vi "Avg_Example_IMAQ.vi"() -> ()   [LabVIEW 2019]
doc: "This example shows how to continously compute and show an averaged image.\nHere the camera class is operated in sequence mode and the required number of images also defines the number of images that will be averaged\nIt is a good starting point for writing own applications.\nBut it will not be fail save, i.e. doesnt react on errors, just handles them forward to the end\n\nUsage:\nSelect your required image count you want to average over before you start the program.\nOnce started, the camera class will be initialized and image record will start automatically.\nInside the acquisition loop the program will record the image sequence.\nThen it calculates the average image and shows it.\nBy using the ROI parameters you can crop the image to select certain regions\n\nBy clicking Quit Application the record will stop and will force an exit of the camera class"
uses:
  camera/Camera.lvclass
panel:
  out "rawImage":u16[][](array[numeric])
  out "Image":T1(plugin-control)
  in  "data_format":T2(ring)=enum."Mono16"
  out "Recorded Images":u32
  in  "Quit":bool
  in  "cropY1":u64=2 min=2 max=1040 step=1
  in  "cropX1":u64=2 min=2 max=1392 step=1
  in  "cropY0":u64=1 min=1 max=1039 step=1
  in  "cropX0":u64=1 min=1 max=1391 step=1
  out "Image Height":u64
  out "Image Width":u64
  in  "dwImgCount":u32=10 caption="Required Number of Images" max=4023
  out "Error":errorcluster {"code" format="%x"}
  # "This example shows how to continously compute and show an averaged image.\nHere the camera class is operated in sequence mode and the required number of images also defines the number of images that will be averaged\nIt is a good starting point for writing own applications.\nBut it will not be fail save, i.e. doesnt react on errors, just handles them forward to the end\n\nUsage:\nSelect your required image count you want to average over before you start the program.\nOnce started, the camera class will be initialized and image record will start automatically.\nInside the acquisition loop the program will record the image sequence.\nThen it calculates the average image and shows it.\nBy using the crop parameters you can crop the image to select certain regions\n\nBy clicking Quit Application the record will stop and will force an exit of the camera class"
  # "pco.labview"
  # "Camera Setup"
  # "Recording Control"
  # "Parameters for image readout"
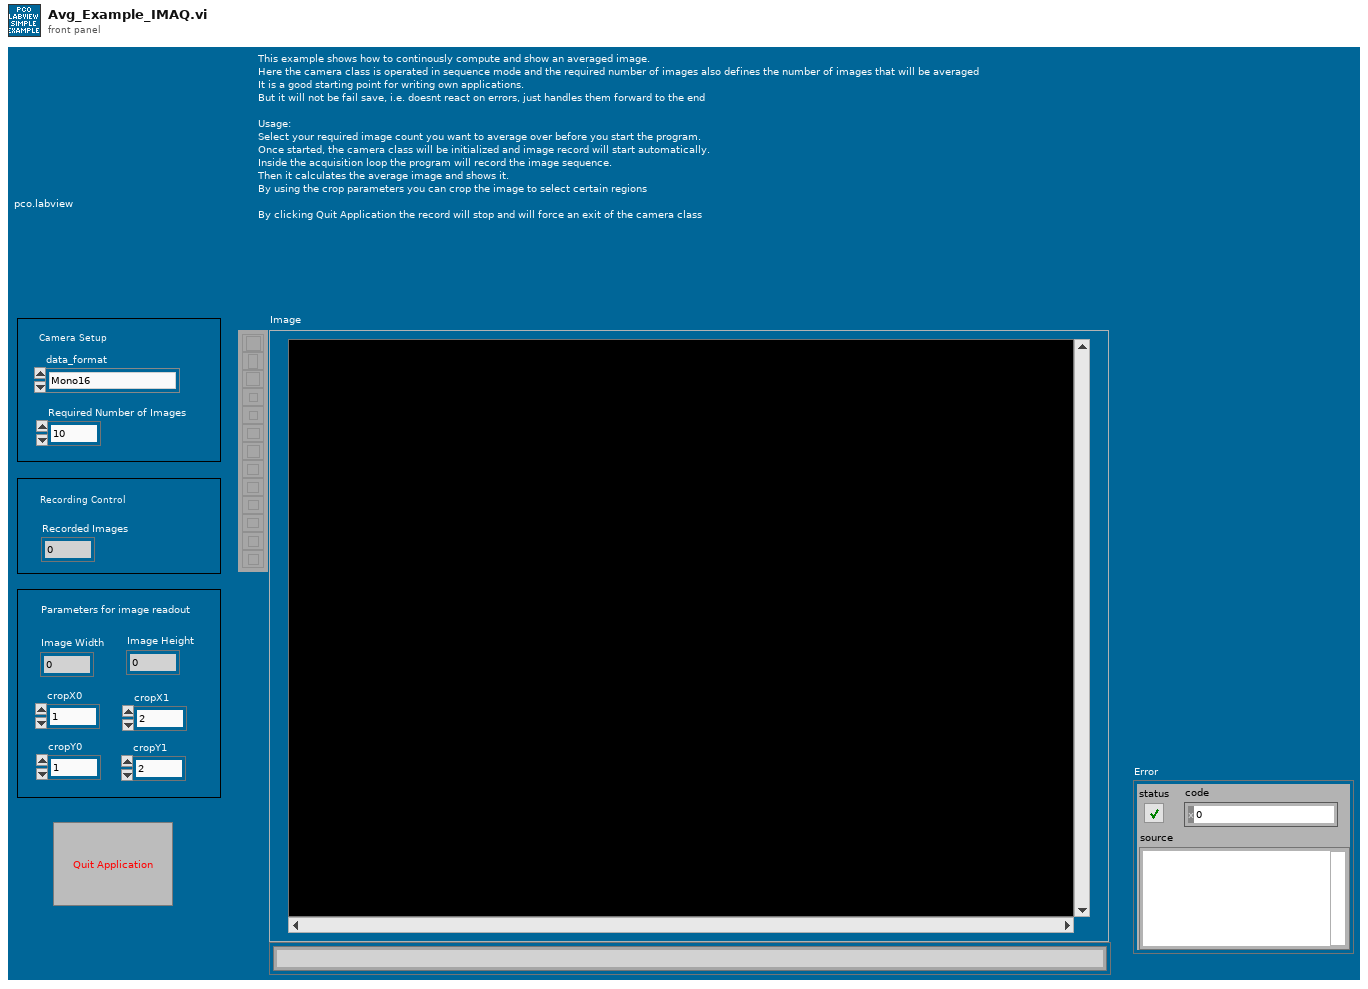
[diagram p1: front panel]
types:
  T1 = typedef "IMAQ Image.ctl" = refnum<image>
  T2 = enum16{"Undefined", "Mono8", "Mono16", "BGRA8", "RGBA8", "BGRA16", "RGBA16", "CompressedMono8"}
  T3 = enum8{"Enabled", "Disabled", "Disabled and Grayed Out"}
  T4 = enum16{"sequence", "sequence non blocking", "ring buffer", "fifo", "tif", "multitif", "pcoraw", "b16", "dicom", "multidicom", "camram_ring", "camram_segment"}
  T5 = cluster{"serial":u32, "type":u16, "sub_type":u16, "interface_type":u16, "bit_resolution":u16, "min_exposure_time_s":dbl, "max_exposure_time_s":dbl, "min_exposure_step_s":dbl, "min_delay_time_s":dbl, "max_delay_time_s":dbl, "min_delay_step_s":dbl, "min_width":u64, "min_height":u64, "max_width":u64, "max_height":u64, "roi_step_horz":u64, "roi_step_vert":u64, "roi_symmetric_horz":bool, "roi_symmetric_vert":bool, "has_timestamp_mode":bool, "has_timestamp_mode_ascii_only":bool, "pixelrate_vec":u32[], "conversion_factor_vec":sgl[], "has_trigger_mode_extexpctrl":bool, "has_acquire_mode":bool, "has_ext_acquire_mode":bool, "has_metadata_mode":bool, "has_ram":bool, "binning_horz_vec":u16[], "binning_vert_vec":u16[], "has_average_binning":bool, "pixel_format_vec":u32[]}
  T6 = typedef "Image Type" = u32
  T7 = typedef "Camera.lvclass/binning.ctl" = cluster{"vert":u16, "horz":u16, "mode":u16}
  T8 = cluster{"exposure_time_s":dbl, "delay_time_s":dbl, "roi":cluster{"x0":u64, "y0":u64, "x1":u64, "y1":u64}, "timestamp_mode":u16, "pixelrate":u32, "conversion_factor":sgl, "trigger_mode":u16, "acquire_mode":u16, "acquire_sequence_number":u32, "metadata_mode":u16, "noisefilter_mode":u16, "pixel_format":u32, "binning":T7, "auto_exposure":cluster{"region":u16, "min_exposure_s":dbl, "max_exposure_s":dbl}}
  T9 = cluster{"Plane 4 (alpha)":u16, "Plane 1 (Red)":u16, "Plane 2 (Green)":u16, "Plane 3 (Blue)":u16}[][]
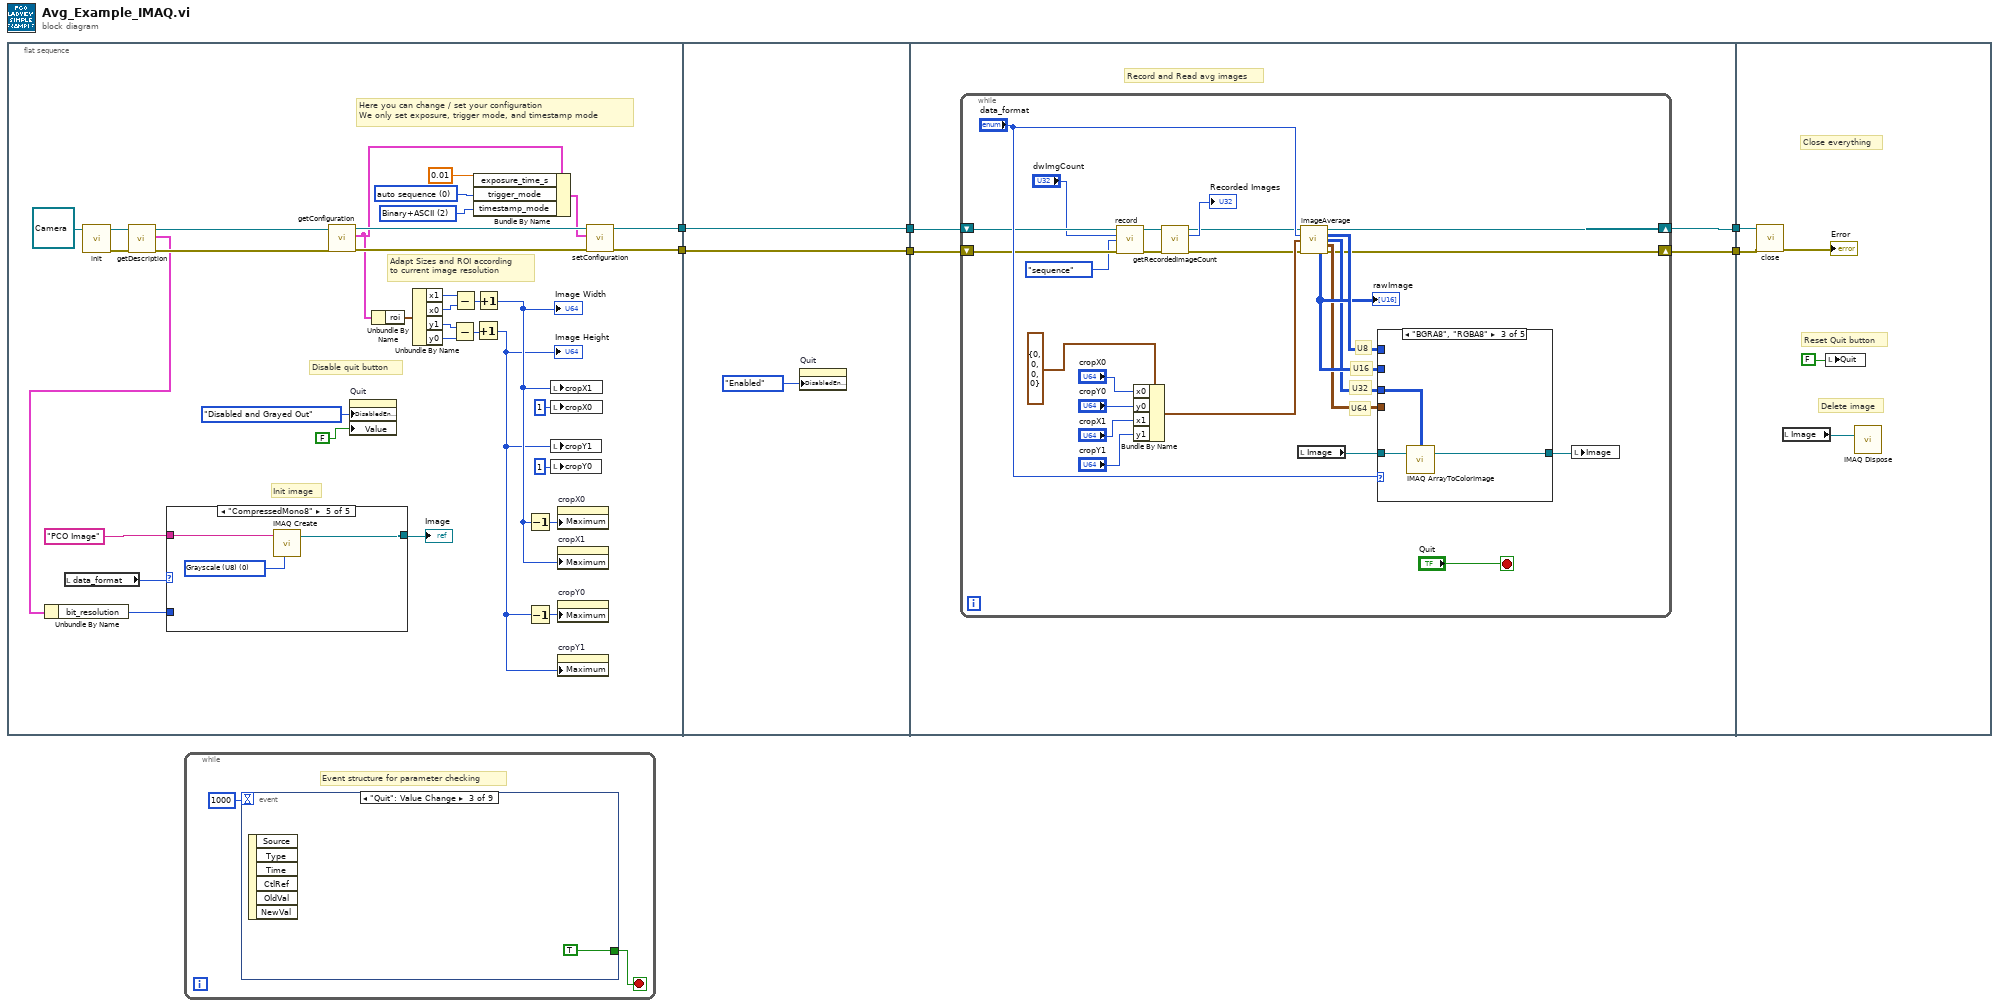
[diagram p0: block diagram]
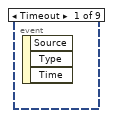
[diagram p2: hidden frame]
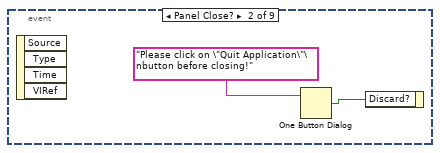
[diagram p3: hidden frame]
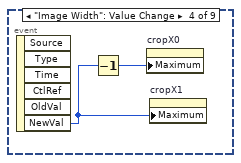
[diagram p4: hidden frame]
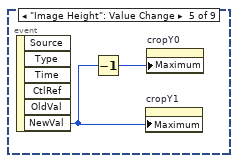
[diagram p5: hidden frame]
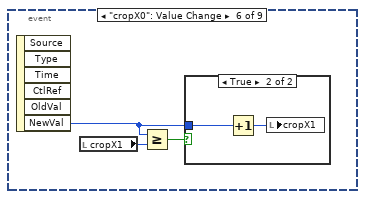
[diagram p6: hidden frame]
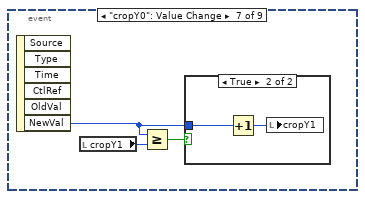
[diagram p8: hidden frame]
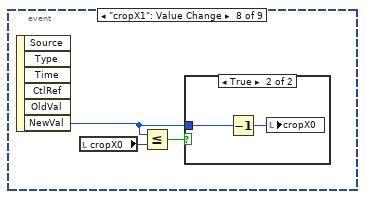
[diagram p10: hidden frame]
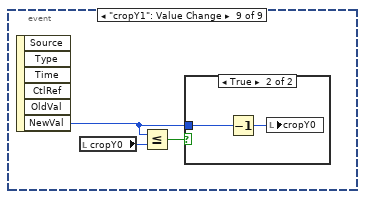
[diagram p12: hidden frame]
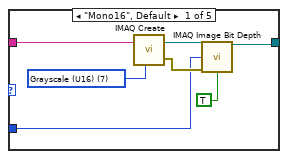
[diagram p14: hidden frame]
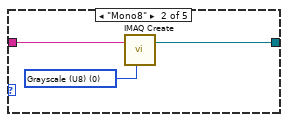
[diagram p15: hidden frame]
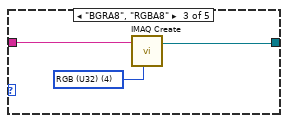
[diagram p16: hidden frame]
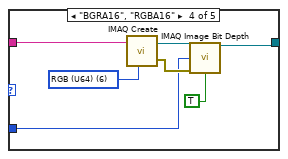
[diagram p17: hidden frame]
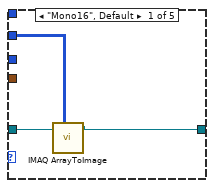
[diagram p18: hidden frame]
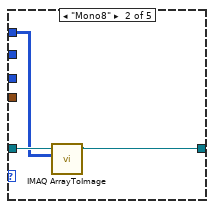
[diagram p19: hidden frame]
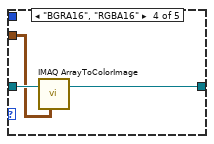
[diagram p20: hidden frame]
diagram:
  n1 = flat-sequence {
    tunnel: [w15] -> w6
    tunnel: [w14] -> w5
    tunnel: w6 -> [w65]
    tunnel: w5 -> [w64]
    tunnel: [w65] -> w4
    tunnel: [w64] -> w3
    tunnel: [w70] -> w2
    tunnel: [w69] -> w1
    tunnel: w3 -> [w68]
    tunnel: w4 -> [w67]
    tunnel: w2 -> [w113]
    tunnel: w1 -> [w112]
    frame #0 {
      w21 = u16 2 items=["OFF", "Binary", "Binary+ASCII", "ASCII"] ("TimestampMode")
      w39 = u16 0 items=["auto sequence"=0, "software trigger"=1, "external exposure start & software trigger"=2, "external exposure control"=3, "external synchronized"=4, "fast external exposure control"=5, "external CDS control"=6, "slow external exposure control"=7, "external synchronized HDSDI"=258] ("TriggerMode")
      # "Here you can change / set your configuration\nWe only set exposure, trigger mode, and timestamp mode"
      # "Init image"
      # "Adapt Sizes and ROI according\nto current image resolution"
      # "Disable quit button"
      n2 = local read "data_format"() -> (w18:T2)
      n3 = call-dynamic "init.vi"("Camera in"=refnum<class "Camera.lvclass"> refnum ("PCOCamera in")) -> ("Camera out"=w12:refnum<class "Camera.lvclass">, "error out"=w13:errorcluster)  [unwired: 8 in]
      n4 = call-dynamic "getDescription.vi"("error in (no error)"=w13, "Camera in"=w12) -> ("error out"=w10:errorcluster, "description"=w9:T5, "Camera out"=w11:refnum<class "Camera.lvclass">)  [unwired: 7 in]
      n5 = Unbundle By Name(w9) -> ("bit_resolution"=w8:u16)
      n6 = case shown="\"CompressedMono8\"" w18 {
        tunnel: "PCO Image" ("Image Name") -> [w46 w50 w52 w59 w62]
        tunnel: [w42 w48 w51 w55 w61] -> w17
        tunnel: w8 -> [w41 _ _ w54 _]
        frame "Mono16", Default {
          w47 = T6 7 items=["Grayscale (U8)", "Grayscale (I16)", "Grayscale (SGL)", "Complex (CSG)", "RGB (U32)", "HSL (U32)", "RGB (U64)", "Grayscale (U16)"] ("Image Type")
          n7 = call "IMAQ Create"("Image Name"=w46, "Image Type"=w47) -> ("New Image"=w44:T1, "error out"=w43:errorcluster)  [unwired: 3 in]
          n8 = call "IMAQ Image Bit Depth"("Image"=w44, "Bit Depth (0)"=w41, "error in (no error)"=w43, "Get/Set Bit Depth? (Set)"=TRUE) -> ("Image Out"=w42:T1)  [unwired: 9 in, 2 out]
        }
        frame "Mono8" {
          w49 = T6 0 items=["Grayscale (U8)", "Grayscale (I16)", "Grayscale (SGL)", "Complex (CSG)", "RGB (U32)", "HSL (U32)", "RGB (U64)", "Grayscale (U16)"] ("Image Type")
          n9 = call "IMAQ Create"("Image Name"=w50, "Image Type"=w49) -> ("New Image"=w48:T1)  [unwired: 3 in, 1 out]
        }
        frame "BGRA8", "RGBA8" {
          w53 = T6 4 items=["Grayscale (U8)", "Grayscale (I16)", "Grayscale (SGL)", "Complex (CSG)", "RGB (U32)", "HSL (U32)", "RGB (U64)", "Grayscale (U16)"] ("Image Type")
          n10 = call "IMAQ Create"("Image Name"=w52, "Image Type"=w53) -> ("New Image"=w51:T1)  [unwired: 3 in, 1 out]
        }
        frame "BGRA16", "RGBA16" {
          w60 = T6 6 items=["Grayscale (U8)", "Grayscale (I16)", "Grayscale (SGL)", "Complex (CSG)", "RGB (U32)", "HSL (U32)", "RGB (U64)", "Grayscale (U16)"] ("Image Type")
          n11 = call "IMAQ Create"("Image Name"=w59, "Image Type"=w60) -> ("New Image"=w57:T1, "error out"=w56:errorcluster)  [unwired: 3 in]
          n12 = call "IMAQ Image Bit Depth"("Image"=w57, "Bit Depth (0)"=w54, "error in (no error)"=w56, "Get/Set Bit Depth? (Set)"=TRUE) -> ("Image Out"=w55:T1)  [unwired: 9 in, 2 out]
        }
        frame "CompressedMono8" {
          w63 = T6 0 items=["Grayscale (U8)", "Grayscale (I16)", "Grayscale (SGL)", "Complex (CSG)", "RGB (U32)", "HSL (U32)", "RGB (U64)", "Grayscale (U16)"] ("Image Type")
          n13 = call "IMAQ Create"("Image Name"=w62, "Image Type"=w63) -> ("New Image"=w61:T1)  [unwired: 3 in, 1 out]
        }
      }
      "Image" <- w17
      n14 = call-dynamic "getConfiguration.vi"("error in (no error)"=w10, "Camera in"=w11) -> ("error out"=w37:errorcluster, "configuration"=w31:T8, "Camera out"=w38:refnum<class "Camera.lvclass">)  [unwired: 7 in]
      n15 = property on="Quit" class="Bool (strict)"("DisabledEnum"=T3."Disabled and Grayed Out" ("Disabled"), "Value"=FALSE ("Stop")) -> ()  [unwired: 2 in, 2 out]
      n16 = Unbundle By Name(w31) -> ("roi"=w30:cluster{"x0":u64, "y0":u64, "x1":u64, "y1":u64})
      n17 = Unbundle By Name(w30) -> ("x1"=w28:u64, "x0"=w29:u64, "y1"=w26:u64, "y0"=w27:u64)
      n18 = Subtract(x=w26, y=w27) -> (x-y=w24:u64)
      n19 = Subtract(x=w28, y=w29) -> (x-y=w25:u64)
      n20 = Bundle By Name(cluster=w31, "exposure_time_s"=0.01, "trigger_mode"=w39, "timestamp_mode"=w21) -> (w36:T8)
      n21 = Increment(x=w24) -> (x+1=w22:u64)
      "Image Height" <- w22
      n22 = Increment(x=w25) -> (x+1=w23:u64)
      "Image Width" <- w23
      n23 = Decrement(x=w23) -> (x-1=w33:u64)
      n24 = Decrement(x=w22) -> (x-1=w32:u64)
      n25 = local write "cropX1"(w23) -> ()
      n26 = local write "cropX0"(u64 1 ("roiY0")) -> ()
      n27 = local write "cropY1"(w22) -> ()
      n28 = local write "cropY0"(u64 1 ("roiY0")) -> ()
      n29 = property on="cropX0" class="DigNum (strict)"("Maximum"=w33) -> ()  [unwired: 2 in, 2 out]
      n30 = property on="cropX1" class="DigNum (strict)"("Maximum"=w23) -> ()  [unwired: 2 in, 2 out]
      n31 = property on="cropY0" class="DigNum (strict)"("Maximum"=w32) -> ()  [unwired: 2 in, 2 out]
      n32 = property on="cropY1" class="DigNum (strict)"("Maximum"=w22) -> ()  [unwired: 2 in, 2 out]
      n33 = call-dynamic "setConfiguration.vi"("error in (no error)"=w37, "configuration"=w36, "Camera in"=w38) -> ("error out"=w14:errorcluster, "Camera out"=w15:refnum<class "Camera.lvclass">)  [unwired: 7 in]
    }
    frame #1 {
      n34 = property on="Quit" class="Bool (strict)"("DisabledEnum"=T3."Enabled" ("Disabled")) -> ()  [unwired: 2 in, 2 out]
    }
    frame #2 {
      # "Record and Read avg images"
      n35 = while {
        shift-right: [w81] -> w70
        shift-left: w67 -> [w80]
        shift-right: [w72] -> w69
        shift-left: w68 -> [w79]
        stop <- "Quit" stop-if-true
        # "U64"
        # "U32"
        # "U16"
        # "U8"
        n36 = call-dynamic "record.vi"("Camera in"=w80, "num_images"="dwImgCount", "record_mode"=T4."sequence", "error in (no error)"=w79) -> ("Camera out"=w78:refnum<class "Camera.lvclass">, "error out"=w77:errorcluster)  [unwired: 10 in]
        n37 = Bundle By Name(cluster=cluster{"x0":u64, "y0":u64, "x1":u64, "y1":u64} {"x0"=0, "y0"=0, "x1"=0, "y1"=0} ("roi"), "x0"="cropX0", "y0"="cropY0", "x1"="cropX1", "y1"="cropY1") -> (w91:cluster{"x0":u64, "y0":u64, "x1":u64, "y1":u64})
        n38 = call-dynamic "getRecordedImageCount.vi"("Camera in"=w78, "error in (no error)"=w77) -> ("Camera out"=w75:refnum<class "Camera.lvclass">, "recorded_image_count"=→"Recorded Images":u32, "error out"=w74:errorcluster)  [unwired: 11 in]
        n39 = local read "Image"() -> (w85:T1)
        n40 = call-dynamic "imageAverage.vi"("Camera in"=w75, "data_format"="data_format", "crop"=w91, "error in (no error)"=w74) -> ("Camera out"=w81:refnum<class "Camera.lvclass">, "image (U8)"=w89:u8[][], "image (U32)"=w87:u32[][], "image (U64)"=w86:T9, "raw_image (U16)"=w88:u16[][], "error out"=w72:errorcluster)  [unwired: 5 in, 1 out]
        "rawImage" <- w88
        n41 = case shown="\"BGRA8\", \"RGBA8\"" "data_format" {
          tunnel: w85 -> [w98 w101 w104 w107 w110]
          tunnel: [w96 w99 w103 w105 w109] -> w84
          tunnel: w86 -> [_ _ _ w106 _]
          tunnel: w87 -> [_ _ w102 _ _]
          tunnel: w89 -> [_ w100 _ _ w108]
          tunnel: w88 -> [w97 _ _ _ _]
          frame "Mono16", Default {
            n42 = call "IMAQ ArrayToImage"("Image Pixels (U16)"=w97, "Image"=w98) -> ("Image Out"=w96:T1)  [unwired: 8 in, 1 out]
          }
          frame "Mono8" {
            n43 = call "IMAQ ArrayToImage"("Image Pixels (U8)"=w100, "Image"=w101) -> ("Image Out"=w99:T1)  [unwired: 8 in, 1 out]
          }
          frame "BGRA8", "RGBA8" {
            n44 = call "IMAQ ArrayToColorImage"("Image Pixels (U32)"=w102, "Image"=w104) -> ("Image Out"=w103:T1)  [unwired: 3 in, 1 out]
          }
          frame "BGRA16", "RGBA16" {
            n45 = call "IMAQ ArrayToColorImage"("Image"=w107, "Image Pixels (U64)"=w106) -> ("Image Out"=w105:T1)  [unwired: 3 in, 1 out]
          }
          frame "CompressedMono8" {
            n46 = call "IMAQ ArrayToImage"("Image Pixels (U8)"=w108, "Image"=w110) -> ("Image Out"=w109:T1)  [unwired: 8 in, 1 out]
          }
        }
        n47 = local write "Image"(w84) -> ()
      }
    }
    frame #3 {
      # "Delete image"
      # "Reset Quit button"
      # "Close everything"
      n48 = call-dynamic "close.vi"("error in (no error)"=w112, "Camera in"=w113) -> ("error out"=→"Error":errorcluster)  [unwired: 9 in]
      n49 = local read "Image"() -> (w111:T1)
      n50 = local write "Quit"(FALSE ("Stop")) -> ()
      n51 = call "IMAQ Dispose"("Image"=w111) -> ()  [unwired: 5 in, 1 out]
    }
  }
  n52 = while {
    stop <- w116 stop-if-true
    # "Event structure for parameter checking"
    n53 = event shown="[2] \"Quit\": Value Change" {
      selector: _ -> [_ _ _ _ _ _ _ _ _]
      dyn-events: _ -> [_ _ _ _ _ _ _ _ _]
      timeout: 1000 -> [_ _ _ _ _ _ _ _ _]
      tunnel: [_ _ TRUE _ _ _ _ _ _] -> w116
      event Timeout {
        n54 = event-data() -> ()  [unwired: 1 in, 3 out]
      }
      event Panel Close? {
        n55 = event-data() -> ()  [unwired: 1 in, 4 out]
        n56 = One Button Dialog(message="Please click on \"Quit Application\"\nbutton before closing!") -> (true=w118:bool)  [unwired: 1 in]
        n57 = event-data("Discard?"=w118) -> ()  [unwired: 1 in, 1 out]
      }
      event "Quit": Value Change {
        n58 = event-data() -> ()  [unwired: 1 in, 6 out]
      }
      event "Image Width": Value Change {
        n59 = event-data() -> ("NewVal"=w121:u64)  [unwired: 1 in, 5 out]
        n60 = Decrement(x=w121) -> (x-1=w122:u64)
        n61 = property on="cropX0" class="DigNum (strict)"("Maximum"=w122) -> ()  [unwired: 2 in, 2 out]
        n62 = property on="cropX1" class="DigNum (strict)"("Maximum"=w121) -> ()  [unwired: 2 in, 2 out]
      }
      event "Image Height": Value Change {
        n63 = event-data() -> ("NewVal"=w123:u64)  [unwired: 1 in, 5 out]
        n64 = Decrement(x=w123) -> (x-1=w124:u64)
        n65 = property on="cropY1" class="DigNum (strict)"("Maximum"=w123) -> ()  [unwired: 2 in, 2 out]
        n66 = property on="cropY0" class="DigNum (strict)"("Maximum"=w124) -> ()  [unwired: 2 in, 2 out]
      }
      event "cropX0": Value Change {
        n67 = event-data() -> ("NewVal"=w125:u64)  [unwired: 1 in, 5 out]
        n68 = local read "cropX1"() -> (w127:u64)
        n69 = Greater Or Equal?(x=w125, y=w127) -> (x >= y?=w126:bool)
        n70 = case shown="True" w126 {
          tunnel: w125 -> [_ w129]
          frame False {
          }
          frame True {
            n71 = Increment(x=w129) -> (x+1=w128:u64)
            n72 = local write "cropX1"(w128) -> ()
          }
        }
      }
      event "cropY0": Value Change {
        n73 = event-data() -> ("NewVal"=w130:u64)  [unwired: 1 in, 5 out]
        n74 = local read "cropY1"() -> (w132:u64)
        n75 = Greater Or Equal?(x=w130, y=w132) -> (x >= y?=w131:bool)
        n76 = case shown="True" w131 {
          tunnel: w130 -> [_ w134]
          frame False {
          }
          frame True {
            n77 = Increment(x=w134) -> (x+1=w133:u64)
            n78 = local write "cropY1"(w133) -> ()
          }
        }
      }
      event "cropX1": Value Change {
        n79 = event-data() -> ("NewVal"=w135:u64)  [unwired: 1 in, 5 out]
        n80 = local read "cropX0"() -> (w137:u64)
        n81 = Less Or Equal?(x=w135, y=w137) -> (x <= y?=w136:bool)
        n82 = case shown="True" w136 {
          tunnel: w135 -> [_ w139]
          frame False {
          }
          frame True {
            n83 = Decrement(x=w139) -> (x-1=w138:u64)
            n84 = local write "cropX0"(w138) -> ()
          }
        }
      }
      event "cropY1": Value Change {
        n85 = event-data() -> ("NewVal"=w140:u64)  [unwired: 1 in, 5 out]
        n86 = local read "cropY0"() -> (w142:u64)
        n87 = Less Or Equal?(x=w140, y=w142) -> (x <= y?=w141:bool)
        n88 = case shown="True" w141 {
          tunnel: w140 -> [_ w144]
          frame False {
          }
          frame True {
            n89 = Decrement(x=w144) -> (x-1=w143:u64)
            n90 = local write "cropY0"(w143) -> ()
          }
        }
      }
    }
  }
